vi "Write configuration.vi"(8 "error in (no error)":errorcluster, 10 "configuration":refnum<class "CEF_serializable configuration.lvclass">, 11 "PS Instrument":refnum<class "Power Supply Instrument.lvclass">) -> (0 "error out":errorcluster, 3 "PS Instrument out":refnum<class "Power Supply Instrument.lvclass">)   [LabVIEW 2025, in "Power Supply.lvlib" / "Power Supply Instrument.lvclass"]
uses:
  Power Supply Instrument.lvclass
  Users/Public/Documents/Sandia National Labs/TSS Plugin/CEF.lvlibp/serializable configuration/CEF_serializable configuration.lvclass
  Users/Public/Documents/Sandia National Labs/TSS Plugin/Abstract Engine.lvlibp/Instrument configuration/Instrument configuration.lvclass
  Power Supply Instrument.lvclass/Power Supply Instrument.ctl
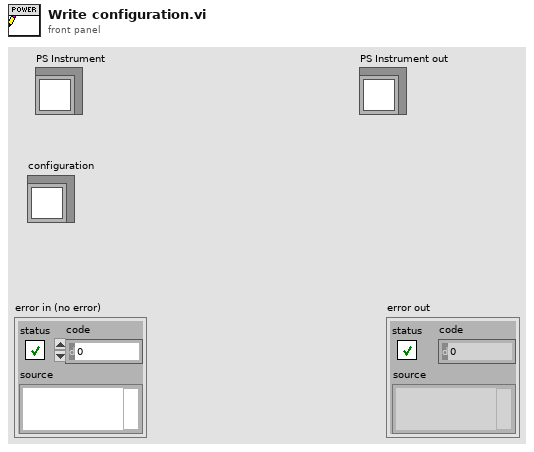
[diagram p1: front panel]
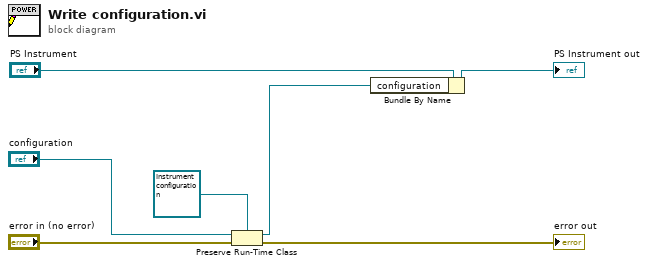
[diagram p0: block diagram]
diagram:
  n1 = Preserve Run-Time Class(object in="configuration", error in="error in (no error)", 2:refnum<class "Instrument configuration.lvclass"> refnum ("Abstract PlugIn.lvlibp:Instrument configuration")) -> (object out=w4:refnum<class "Instrument configuration.lvclass">, error out=→"error out":errorcluster)
  n2 = Bundle By Name(cluster="PS Instrument", "configuration"=w4) -> (→"PS Instrument out":refnum<class "Power Supply Instrument.lvclass">)
